vi "Group Count.vi"(8 "error in (no error)":errorcluster, 11 "Runtime Configuration in":refnum<class "Core Configuration.lvclass">) -> (0 "error out":errorcluster, 2 "group count":i32, 3 "Runtime Configuration out":refnum<class "Core Configuration.lvclass">)   [LabVIEW 2021, in "DSF Core.lvlib" / "Core Configuration.lvclass"]
uses:
  Core Configuration.lvclass
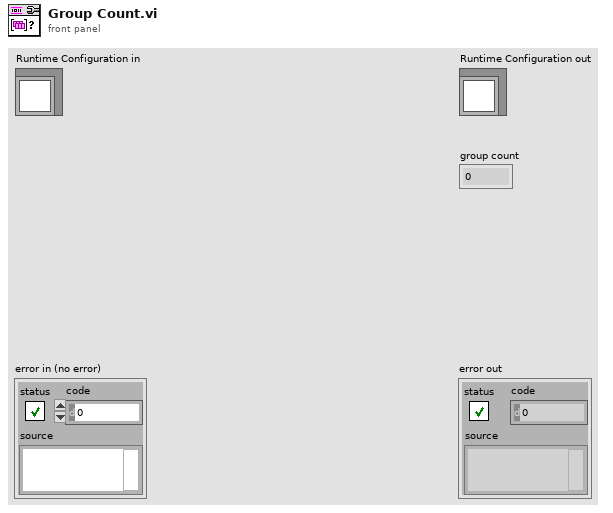
[diagram p1: front panel]
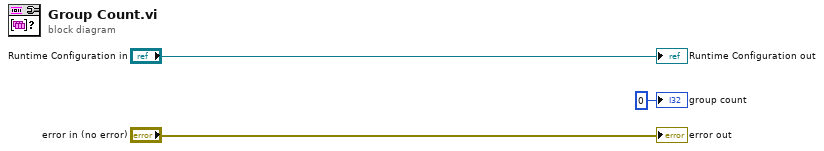
[diagram p0: block diagram]
diagram:
  "error out" <- "error in (no error)"
  "Runtime Configuration out" <- "Runtime Configuration in"
  "group count" <- 0 ("group count")
